vi "ActBalance.vi"(10 "MaxSpeed (ft/s)":dbl) -> (1 "XSpeedDemand":dbl, 3 "Done":bool)   [LabVIEW 2020]
doc: "Robot begins balancing towards the \"GyroZero\" position. \n\nInputs:\n-- MaxSpeed -- Double -- in ft/s, the MaxSpeed the robot can go (Has no effect above 1.5)\n\n\nOutputs:\n-- Done -- Bool -- has the robot reached its target distance\n-- LeftSpeedDemand -- Double -- Speed Demand for left drive train inorder to reach target -- \n-- RightSpeedDemand -- Double -- Speed Demand for left drive train inorder to reach target --"
uses:
  <vilib>/Rock Robotics/WPI/ThirdParty/JAS_Junk/TrajLib/VI/Util_GetTime_U32.vi
  <vilib>/Rock Robotics/WPI/ThirdParty/JAS_Junk/TrajLib/LinearFilter_ResetToValue.vi
  <vilib>/Rock Robotics/WPI/ThirdParty/JAS_Junk/TrajLib/LinearFilter_Calculate.vi
  <vilib>/Rock Robotics/WPI/ThirdParty/JAS_Junk/TrajLib/Timer_New.vi
  <vilib>/Rock Robotics/SystemInterfaces/Utilities/FPGA_UtilitiesRead LocalTime.vi
  <vilib>/Rock Robotics/WPI/ThirdParty/JAS_Junk/TrajLib/VI/Util_GetTime_U64.vi
  <vilib>/Rock Robotics/Network Tables/NT Write Number.vi
  <vilib>/Rock Robotics/WPI/ThirdParty/JAS_Junk/TrajLib/LinearFilter_MovingAverage.vi
  <vilib>/Rock Robotics/WPI/ThirdParty/JAS_Junk/TrajLib/LinearFilter_LowPassBW1.vi
  <vilib>/Rock Robotics/WPI/ThirdParty/JAS_Junk/TrajLib/LinearFilter_LowPassBW2.vi
  <vilib>/Rock Robotics/WPI/ThirdParty/JAS_Junk/TrajLib/LinearFilter_HighPassBW1.vi
  <vilib>/Rock Robotics/WPI/ThirdParty/JAS_Junk/TrajLib/LinearFilter_HighPassBW2.vi
  <vilib>/Utility/semaphor.llb/Obtain Semaphore Reference.vi
  <vilib>/Rock Robotics/WPI/ThirdParty/JAS_Junk/TrajLib/Timer_Reset.vi
  <vilib>/Rock Robotics/WPI/ThirdParty/JAS_Junk/TrajLib/Timer_Start.vi
  <vilib>/Rock Robotics/WPI/ThirdParty/JAS_Junk/TrajLib/Timer_Stop.vi
  <vilib>/Rock Robotics/WPI/ThirdParty/JAS_Junk/TrajLib/Timer_HasPeriodPassedOnce.vi
  <vilib>/Rock Robotics/WPI/ThirdParty/JAS_Junk/TrajLib/Trajectory_Library.lvlib
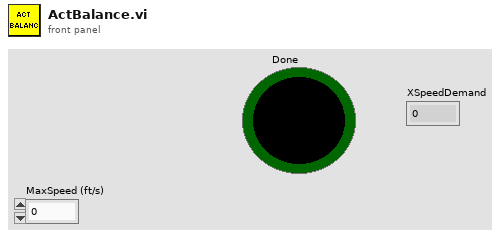
[diagram p1: front panel]
types:
  T1 = enum16{"Moving Average", "Low Pass 1st Order Butterworth", "Low Pass 2nd Order Butterworth", "High Pass 1st Order Butterworth", "High Pass 2nd Order Butterworth"}
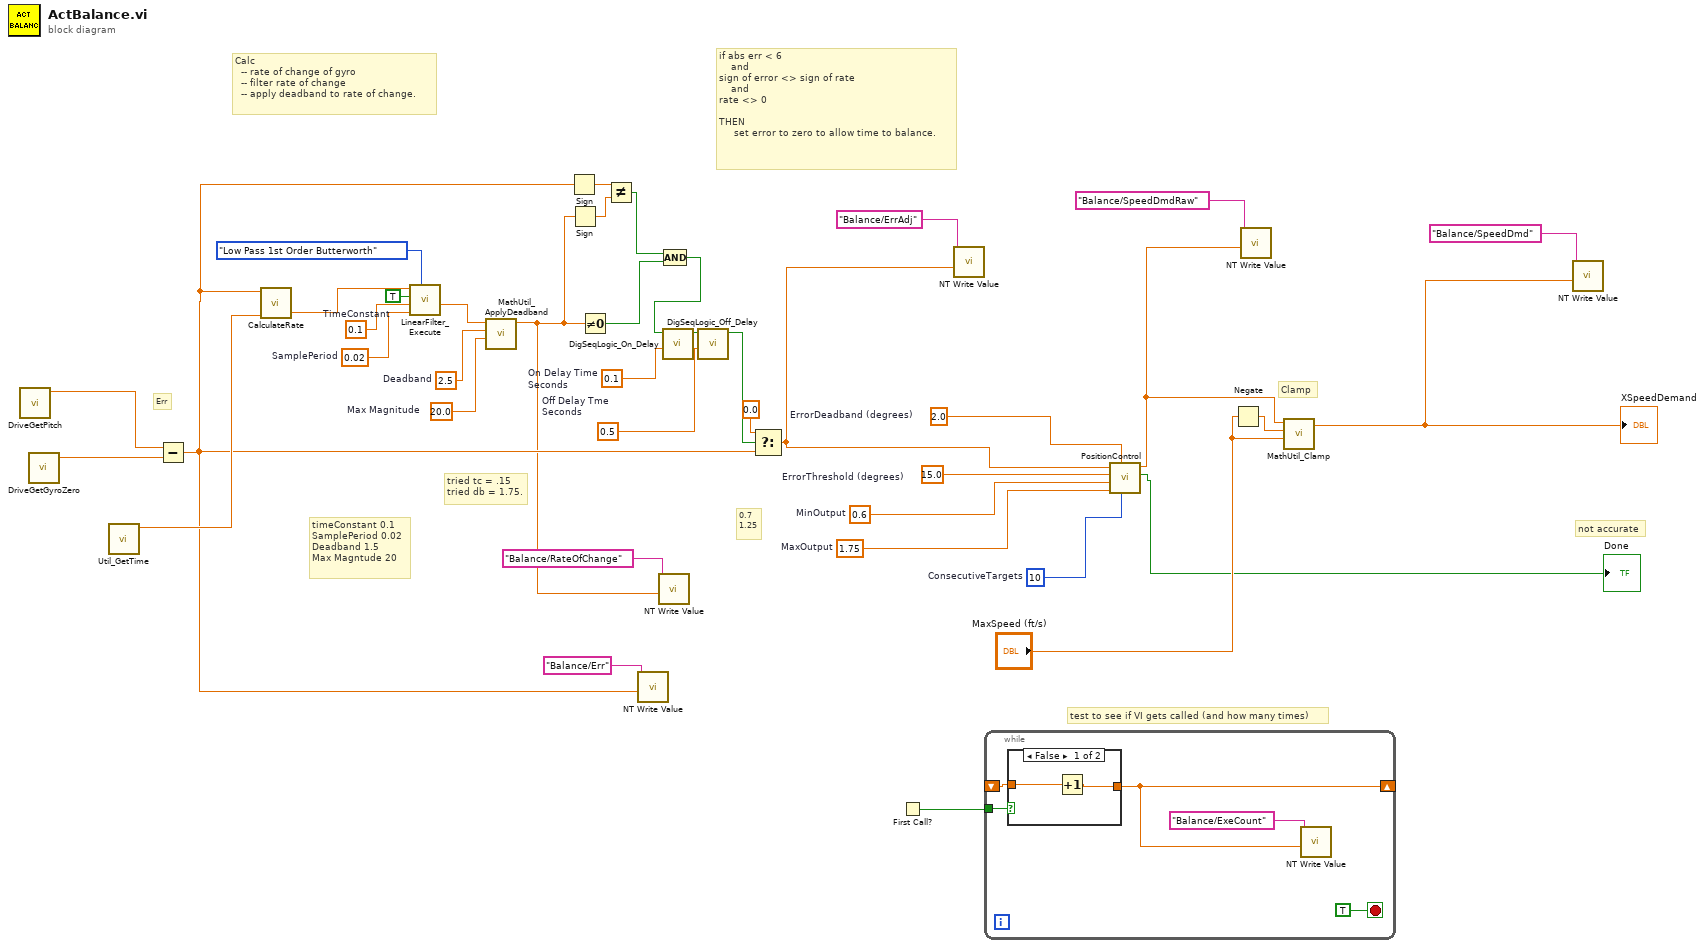
[diagram p0: block diagram]
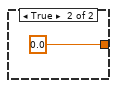
[diagram p2: hidden frame]
diagram:
  w3 = 0.5  # Off Delay Tme Seconds
  w5 = 0.1  # On Delay Time Seconds
  w24 = 0.02  # SamplePeriod
  w23 = 0.1  # TimeConstant
  w25 = 20.0  # Max Magnitude
  w26 = 2.5  # Deadband
  w35 = 1.75  # MaxOutput
  w36 = 0.6  # MinOutput
  w34 = 10  # ConsecutiveTargets
  w39 = 2.0  # ErrorDeadband (degrees)
  w40 = 15.0  # ErrorThreshold (degrees)
  # "test to see if VI gets called (and how many times)"
  # "not accurate"
  # "if abs err < 6 \n    and\nsign of error <> sign of rate\n    and\nrate <> 0\n\nTHEN\n     set error to zero to allow time to balance."
  # "tried tc = .15\ntried db = 1.75."
  # "Calc\n  -- rate of change of gyro\n  -- filter rate of change\n  -- apply deadband to rate of change."
  # "Err"
  # "0.7\n1.25"
  # "timeConstant 0.1\nSamplePeriod 0.02\nDeadband 1.5\nMax Magntude 20"
  # "Clamp"
  n1 = call "DriveGetPitch.vi"() -> ("Pitch"=w32:dbl)  [unwired: 11 in]
  n2 = call "DriveGetGyroZero.vi"() -> ("GyroZero"=w33:dbl)  [unwired: 11 in]
  n3 = call <vilib>:"Util_GetTime.vi"() -> ("FPGA_Time_Seconds"=w27:dbl)  [unwired: 9 in, 2 out]
  n4 = Subtract(x=w32, y=w33) -> (x-y=w16:dbl)
  n5 = call "CalculateRate.vi"("Time (s)"=w27, "Distance (units)"=w16) -> ("Rate (units/s)"=w19:dbl)  [unwired: 9 in]
  n6 = call <vilib>:"LinearFilter_Execute.vi"("Filter Type"=T1."Low Pass 1st Order Butterworth", "SamplePeriod"=w24, "TimeConstant"=w23, "Enable"=TRUE, "Input"=w19) -> ("Output"=w18:dbl)  [unwired: 5 in, 1 out]
  n7 = call <vilib>:"MathUtil_ApplyDeadband.vi"("Max Magnitude"=w25, "Deadband"=w26, "Value"=w18) -> ("Result"=w7:dbl)  [unwired: 8 in]
  n8 = Sign(1:w16) -> (0:w30:dbl)
  n9 = Sign(1:w7) -> (0:w29:dbl)
  n10 = Not Equal To 0?(x=w7) -> (x != 0?=w20:bool)
  n11 = Not Equal?(x=w30, y=w29) -> (x != y?=w28:bool)
  n12 = call-poly <vilib>:"NT Write Value.vi"("value"=w16, "name"="Balance/Err") -> ()  [unwired: 9 in, 1 out]
  n13 = call-poly <vilib>:"NT Write Value.vi"("value"=w7, "name"="Balance/RateOfChange") -> ()  [unwired: 9 in, 1 out]
  n14 = Compound Arithmetic op=AND(w28, w20) -> (w4:bool)
  n15 = call <vilib>:"DigSeqLogic_On_Delay.vi"("Delay"=w5, "Input"=w4) -> ("Output"=w2:bool)  [unwired: 8 in, 1 out]
  n16 = call <vilib>:"DigSeqLogic_Off_Delay.vi"("Delay"=w3, "Input"=w2) -> ("Output"=w1:bool)  [unwired: 8 in, 1 out]
  n17 = Select(t=0.0, s=w1, f=w16) -> (s? t:f=w14:dbl)
  n18 = First Call?() -> (First Call?: T/F=w9:bool)
  n19 = call-poly <vilib>:"NT Write Value.vi"("value"=w14, "name"="Balance/ErrAdj") -> ()  [unwired: 9 in, 1 out]
  n20 = while {
    tunnel: w9 -> [w44]
    shift-right: [w41] -> _
    shift-left: _ -> [w43]
    stop <- TRUE stop-if-true
    n21 = case shown="False" w44 {
      tunnel: [w47 0.0] -> w41
      tunnel: w43 -> [w46 _]
      frame False {
        n22 = Increment(x=w46) -> (x+1=w47:dbl)
      }
      frame True {
      }
    }
    n23 = call-poly <vilib>:"NT Write Value.vi"("value"=w41, "name"="Balance/ExeCount") -> ()  [unwired: 9 in, 1 out]
  }
  n24 = call "PositionControl.vi"("ConsecutiveTargets"=w34, "ErrorDeadband"=w39, "MaxOutput"=w35, "MinOutput"=w36, "ErrorThreshold"=w40, "Error"=w14) -> ("OnTarget"=→"Done":bool, "OutputValue"=w12:dbl)  [unwired: 3 in, 1 out]
  n25 = Negate(x="MaxSpeed (ft/s)") -> (-x=w38:dbl)
  n26 = call-poly <vilib>:"NT Write Value.vi"("value"=w12, "name"="Balance/SpeedDmdRaw") -> ()  [unwired: 9 in, 1 out]
  n27 = call <vilib>:"MathUtil_Clamp.vi"("High Limit"="MaxSpeed (ft/s)", "Low Limit"=w38, "Value"=w12) -> ("Result"=w10:dbl)  [unwired: 8 in]
  "XSpeedDemand" <- w10
  n28 = call-poly <vilib>:"NT Write Value.vi"("value"=w10, "name"="Balance/SpeedDmd") -> ()  [unwired: 9 in, 1 out]
